vi "NI6071E.ProcCases.vi"(0 "i ref in":refnum<vi>, 1 "selector":string, 2 "data":i8[](array[numeric]), 3 "call cluster":T4={"Object"="", "Selector"="", "CallType"=enum."synchronous", "Async Object"="", "Async Selector"="", "Data Descriptor"="", "Data"=[], "Error #"=0, "Expire"=0}, 5 "error in":errorcluster) -> (14 "i ref out":refnum<vi>, 17 "answer cluster":T4={"Object"="", "Selector"="", "CallType"=enum."synchronous", "Async Object"="", "Async Selector"="", "Data Descriptor"="", "Data"=[], "Error #"=0, "Expire"=0}, 19 "error out":errorcluster)   [LabVIEW 2014, in "NI6071E.lvlib"]
doc: "This method is called by a process from within the default case in the event loop. The methods of a class that are linked to events will be called from THIS method. Add your code here."
uses:
  NI6071E.lvlib
  CSCore/CSSystem/CoreDefs/CoreDefs.call_type.ctl
  CSCore/BaseProcess/BaseProcess.descriptor string definition.ctl
  CSCore/CSSystem/CoreDefs/CoreDefs.rawDataType.ctl
  NI6071EConfig.ctl
  NI6071EStart.ctl
  NI6071ERead.ctl
  CSCore/CSSystem/CoreLib/CoreLib.byte array 2 string.vi
  CSCore/CSSystem/CoreLib/CoreLib.byte array 2 int.vi
  CSCore/CSSystem/CoreLib/CoreLib.string 2 byte array.vi
  CSCore/BaseProcess/BaseProcess.lvlib
  CSCore/CSSystem/CoreLib/CoreLib.lvlib
panel:
  in  "NI6071E Read":T1={"time limit in sec (-1:auto calculate)"=-1.0, "number of scans to read (-1:all)"=-1} {"time limit in sec (-1:auto calculate)" format="%0.2f"}
  in  "NI6071E Start":T2={"scan rate (40000 scans/sec)"=1000.0, "trigger type (analog)"=enum."no trigger", "edge or slope \n(rising)"=enum."rising", "number of buffers to acquire (1)"=1, "analog chan (PFI0) & level (2.00)"={"trigger channel (empty)"="", "level (0.0)"=0.0}, "[additional trig params]"={"hysteresis (0.0)"=-1.0, "coupling (no change:0)"=enum."no change", "delay (0 sec)"=0.0, "skip count (0)"=0, "time limit (0 sec)"=0.0}} {"[additional trig params]"."time limit (0 sec)" format="%0.2f"; "[additional trig params]"."delay (0 sec)" format="%0.2f"; "[additional trig params]"."hysteresis (0.0)" format="%0.2f"; "analog chan (PFI0) & level (2.00)"."level (0.0)" format="%0.2f"; "scan rate (40000 scans/sec)" format="%0.2f"}
  in  "NI6071E Config":T3={"device (1)"=5, "channels (0)"=["0", "1", "2"], "buffer size (1000 scans)"=1000, "[number of buffers] (1)"=1, "measurement mode structure"={"measurement mode"=0, "reserved"=0}, "input limits (no change)"=[], "coupling & input config (no change:0)"=[]} {"measurement mode structure"."measurement mode" items=["no change", "Volts", "Volts RMS", "Ohms", "Diode", "4-wire ohms", "Current", "Current RMS"]; "coupling & input config (no change:0)"."input config (no change:0)" items=["no change", "differential", "ref. single-ended", "non-ref. single-ended", "4-wire"]; "input limits (no change)"."low limit (0.0)" format="%0.2f"; "input limits (no change)"."high limit (0.0)" format="%0.2f"}
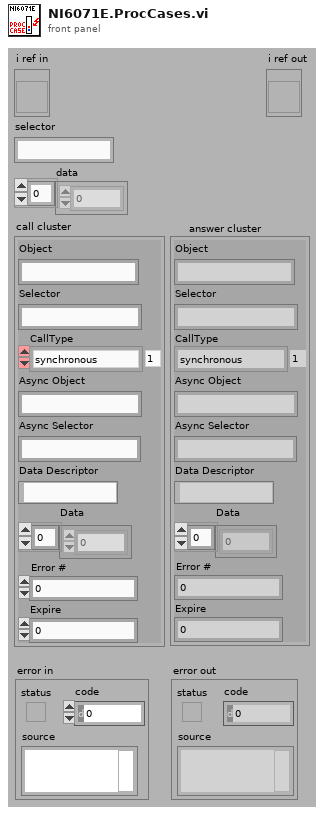
[diagram p1: front panel]
types:
  T1 = typedef "NI6071E.lvlib/NI6071ERead.ctl" = cluster{"time limit in sec (-1:auto calculate)":sgl, "number of scans to read (-1:all)":i32}
  T2 = typedef "NI6071E.lvlib/NI6071EStart.ctl" = cluster{"scan rate (40000 scans/sec)":sgl, "trigger type (analog)":enum16{"no trigger", "analog", "digital A", "digital A & B", "scan clock gate"}, "edge or slope \n(rising)":enum16{"no change", "rising", "falling"}, "number of buffers to acquire (1)":i32, "analog chan (PFI0) & level (2.00)":cluster{"trigger channel (empty)":string, "level (0.0)":sgl}, "[additional trig params]":cluster{"hysteresis (0.0)":sgl, "coupling (no change:0)":enum16{"no change", "DC", "AC"}, "delay (0 sec)":sgl, "skip count (0)":i32, "time limit (0 sec)":sgl}}
  T3 = typedef "NI6071E.lvlib/NI6071EConfig.ctl" = cluster{"device (1)":i16, "channels (0)":tag[], "buffer size (1000 scans)":i32, "[number of buffers] (1)":i32, "measurement mode structure":cluster{"measurement mode":u16, "reserved":u32}, "input limits (no change)":cluster{"high limit (0.0)":sgl, "low limit (0.0)":sgl}[], "coupling & input config (no change:0)":cluster{"coupling (no change:0)":enum16{"no change", "DC", "AC", "GND", "internal ref."}, "input config (no change:0)":u16}[]}
  T4 = typedef "CoreDefs.call_type.ctl" = cluster{"Object":string, "Selector":string, "CallType":enum16{"simple", "synchronous", "asynchronous"}, "Async Object":string, "Async Selector":string, "Data Descriptor":T5, "Data":T6, "Error #":i32, "Expire":u32}
  T5 = typedef "BaseProcess.lvlib/BaseProcess.descriptor string definition.ctl" = string
  T6 = typedef "CoreDefs.rawDataType.ctl" = i8[]
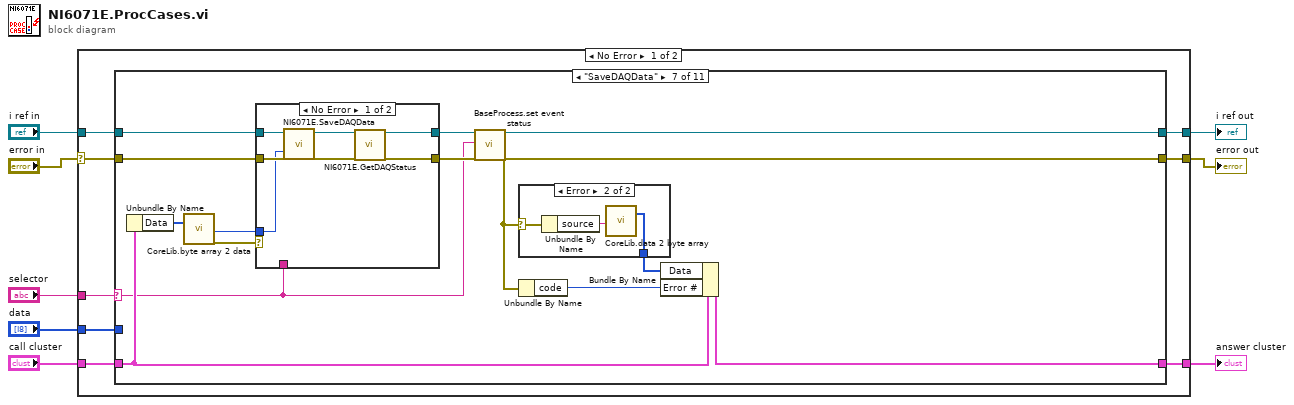
[diagram p0: block diagram]
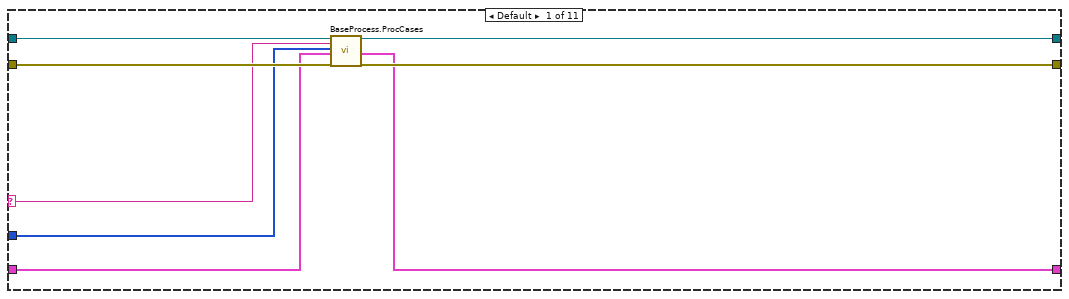
[diagram p2: hidden frame]
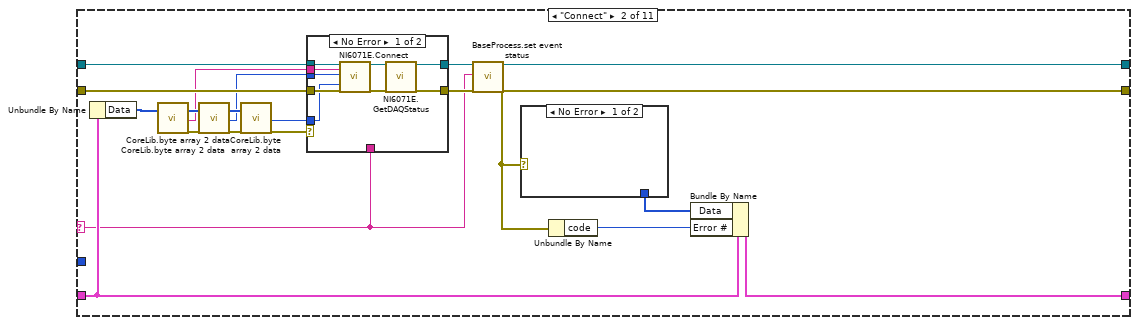
[diagram p3: hidden frame]
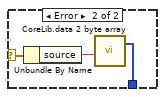
[diagram p4: hidden frame]
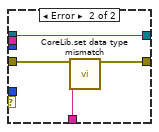
[diagram p5: hidden frame]
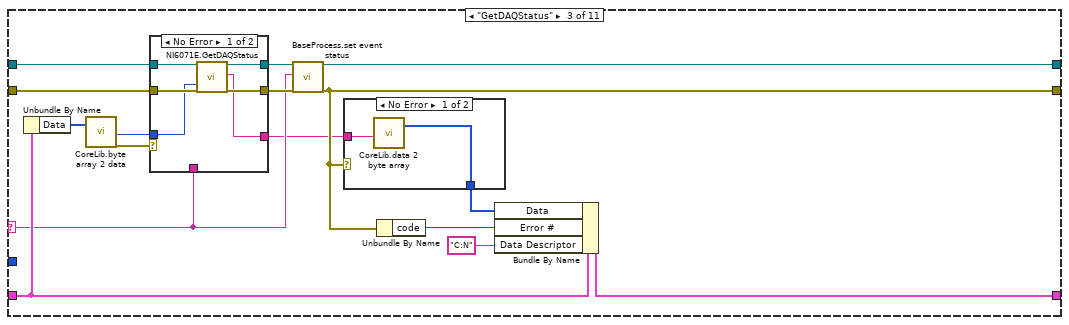
[diagram p6: hidden frame]
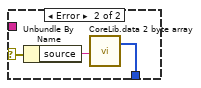
[diagram p7: hidden frame]
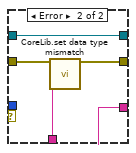
[diagram p8: hidden frame]
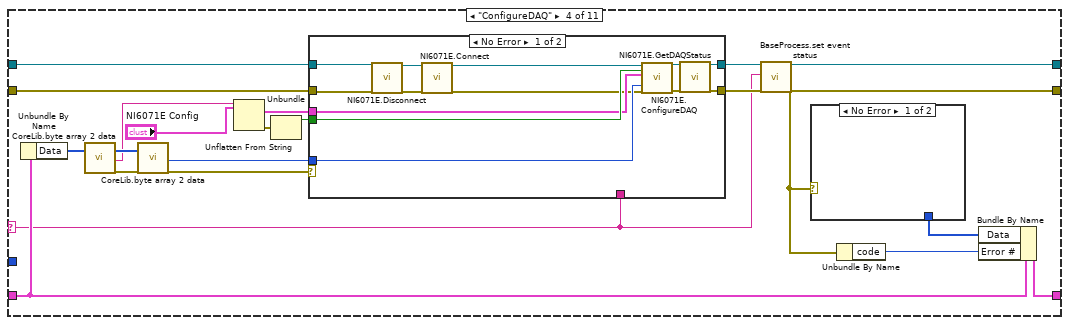
[diagram p9: hidden frame]
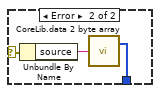
[diagram p10: hidden frame]
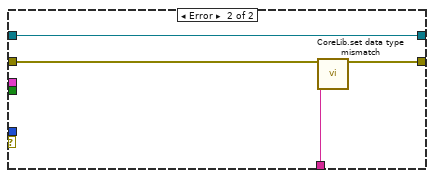
[diagram p11: hidden frame]
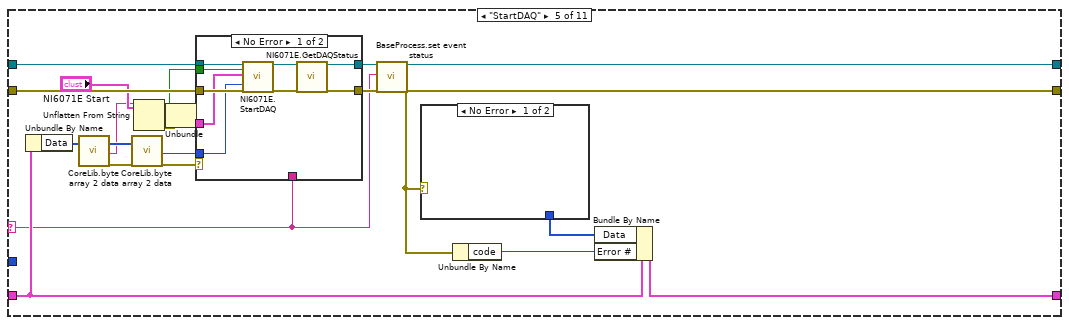
[diagram p12: hidden frame]
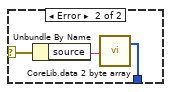
[diagram p13: hidden frame]
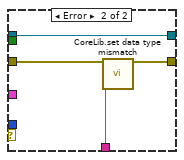
[diagram p14: hidden frame]
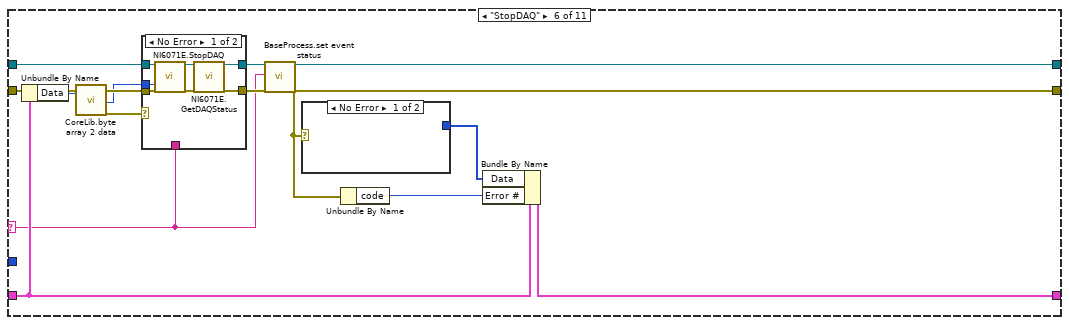
[diagram p15: hidden frame]
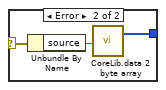
[diagram p16: hidden frame]
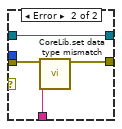
[diagram p17: hidden frame]
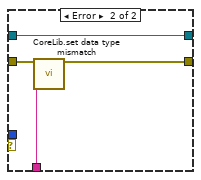
[diagram p19: hidden frame]
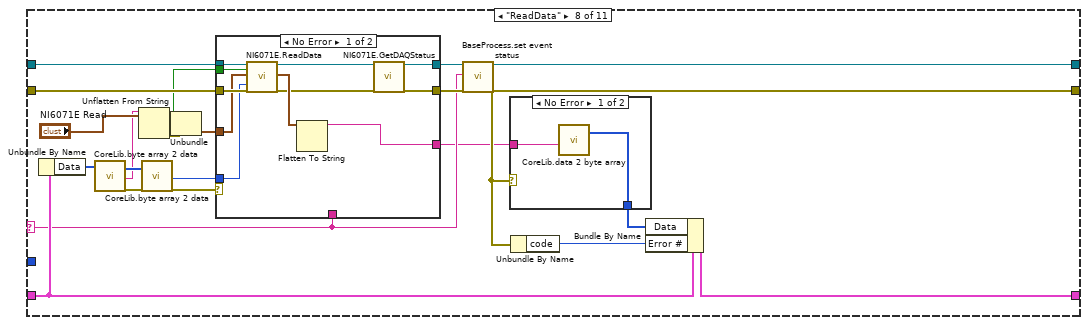
[diagram p20: hidden frame]
diagram:
  n1 = case shown="No Error" "error in" {
    selector: "error in" -> [w9 w352]
    tunnel: "selector" -> [w16 _]
    tunnel: [w15 w353] -> w7
    tunnel: "call cluster" -> [w14 w353]
    tunnel: "i ref in" -> [w13 w354]
    tunnel: [w12 w354] -> w4
    tunnel: [w11 w352] -> w3
    tunnel: "data" -> [w10 _]
    frame No Error {
      n2 = case shown="\"SaveDAQData\"" w16 {
        selector: w16 -> [w19 w36 w68 w105 w146 w176 w204 w240 w276 w310 w339]
        tunnel: w13 -> [w18 w44 w76 w113 w154 w184 w212 w248 w284 w318 w342]
        tunnel: [w24 w35 w67 w104 w145 w175 w203 w239 w275 w309 w344] -> w12
        tunnel: w14 -> [w20 w41 w73 w110 w151 w181 w209 w245 w281 w315 w347]
        tunnel: [w21 w40 w72 w109 w150 w180 w208 w244 w280 w314 w346] -> w15
        tunnel: w9 -> [w23 w43 w75 w112 w153 w183 w211 w247 w283 w317 w341]
        tunnel: [w22 w37 w69 w106 w147 w177 w205 w241 w277 w311 w345] -> w11
        tunnel: w10 -> [w17 _ _ _ _ _ _ _ _ _ _]
        frame Default {
          n3 = call "BaseProcess.ProcCases.vi"("i ref in"=w18, "selector"=w19, "Data"=w17, "call cluster"=w20, "error in (no error)"=w23) -> ("i ref out"=w24:refnum<vi>, "answer cluster"=w21:T4, "error out"=w22:errorcluster)  [unwired: 12 in]
        }
        frame "Connect" {
          n4 = Unbundle By Name(w41) -> ("Data"=w29:T6)
          n5 = call-poly "CoreLib.byte array 2 data.vi"("byteArray"=w29) -> ("byteArray out"=w33:T6, "string"=w28:string, "error out"=w32:errorcluster)  [unwired: 16 in]
          n6 = call-poly "CoreLib.byte array 2 data.vi"("byteArray"=w33, "error in (no error)"=w32) -> ("byteArray out"=w31:T6, "i32"=w27:i32, "error out"=w30:errorcluster)  [unwired: 15 in]
          n7 = call-poly "CoreLib.byte array 2 data.vi"("byteArray"=w31, "error in (no error)"=w30) -> ("i32"=w26:i32, "error out"=w25:errorcluster)  [unwired: 15 in, 1 out]
          n8 = case shown="No Error" w25 {
            tunnel: [w50 w60] -> w39
            tunnel: w44 -> [w55 w60]
            tunnel: w43 -> [w54 w59]
            tunnel: [w48 w58] -> w38
            tunnel: w27 -> [w56 _]
            tunnel: w36 -> [_ w57]
            tunnel: w28 -> [w53 _]
            tunnel: w26 -> [w52 _]
            frame No Error {
              n9 = call "NI6071E.Connect.vi"("i ref in"=w55, "Node name"=w53, "Port"=w56, "timeout ms (60000)"=w52, "error in (no error)"=w54) -> ("i ref out"=w51:refnum<vi>, "error out"=w49:errorcluster)  [unwired: 13 in]
              n10 = call "NI6071E.GetDAQStatus.vi"("i ref in"=w51, "error in (no error)"=w49) -> ("i ref out"=w50:refnum<vi>, "error out"=w48:errorcluster)  [unwired: 15 in, 1 out]
            }
            frame Error {
              n11 = call "CoreLib.set data type mismatch.vi"("error in (no error)"=w59, "error source"=w57) -> ("error out"=w58:errorcluster)  [unwired: 17 in]
            }
          }
          n12 = call "BaseProcess.set event status.vi"("i ref in"=w39, "EventStatus"=w36, "error in (no error)"=w38) -> ("i ref out"=w35:refnum<vi>, "error out"=w37:errorcluster)  [unwired: 14 in, 1 out]
          n13 = case shown="No Error" w37 {
            selector: w37 -> [_ w47]
            tunnel: [_ w45] -> w34
            frame No Error {
            }
            frame Error {
              n14 = Unbundle By Name(w47) -> ("source"=w46:string)
              n15 = call-poly "CoreLib.data 2 byte array.vi"("string"=w46) -> ("byteArray out"=w45:T6)  [unwired: 18 in]
            }
          }
          n16 = Unbundle By Name(w37) -> ("code"=w42:i32)
          n17 = Bundle By Name(cluster=w41, "Data"=w34, "Error #"=w42) -> (w40:T4)
        }
        frame "GetDAQStatus" {
          n18 = Unbundle By Name(w73) -> ("Data"=w63:T6)
          n19 = call-poly "CoreLib.byte array 2 data.vi"("byteArray"=w63) -> ("i32"=w62:i32, "error out"=w61:errorcluster)  [unwired: 16 in, 1 out]
          n20 = case shown="No Error" w61 {
            tunnel: [w86 w92] -> w71
            tunnel: w76 -> [w87 w92]
            tunnel: w75 -> [w85 w91]
            tunnel: [w84 w90] -> w70
            tunnel: w68 -> [_ w89]
            tunnel: w62 -> [w83 _]
            tunnel: [w82 "" ("Status")] -> w65
            frame No Error {
              n21 = call "NI6071E.GetDAQStatus.vi"("i ref in"=w87, "timeout ms (60000)"=w83, "error in (no error)"=w85) -> ("i ref out"=w86:refnum<vi>, "Status"=w82:string, "error out"=w84:errorcluster)  [unwired: 14 in]
            }
            frame Error {
              n22 = call "CoreLib.set data type mismatch.vi"("error in (no error)"=w91, "error source"=w89) -> ("error out"=w90:errorcluster)  [unwired: 17 in]
            }
          }
          n23 = call "BaseProcess.set event status.vi"("i ref in"=w71, "EventStatus"=w68, "error in (no error)"=w70) -> ("i ref out"=w67:refnum<vi>, "error out"=w69:errorcluster)  [unwired: 14 in, 1 out]
          n24 = case shown="No Error" w69 {
            selector: w69 -> [_ w81]
            tunnel: w65 -> [w78 _]
            tunnel: [w77 w79] -> w64
            frame No Error {
              n25 = call-poly "CoreLib.data 2 byte array.vi"("string"=w78) -> ("byteArray out"=w77:T6)  [unwired: 18 in]
            }
            frame Error {
              n26 = Unbundle By Name(w81) -> ("source"=w80:string)
              n27 = call-poly "CoreLib.data 2 byte array.vi"("string"=w80) -> ("byteArray out"=w79:T6)  [unwired: 18 in]
            }
          }
          n28 = Unbundle By Name(w69) -> ("code"=w74:i32)
          n29 = Bundle By Name(cluster=w73, "Data"=w64, "Error #"=w74, "Data Descriptor"="C:N") -> (w72:T4)
        }
        frame "ConfigureDAQ" {
          n30 = Unbundle By Name(w110) -> ("Data"=w96:T6)
          n31 = call-poly "CoreLib.byte array 2 data.vi"("byteArray"=w96) -> ("byteArray out"=w100:T6, "string"=w98:string, "error out"=w99:errorcluster)  [unwired: 16 in]
          n32 = call-poly "CoreLib.byte array 2 data.vi"("byteArray"=w100, "error in (no error)"=w99) -> ("i32"=w97:i32, "error out"=w95:errorcluster)  [unwired: 15 in, 1 out]
          n33 = Unflatten From String(type="NI6071E Config", binary string=w98) -> (value=w102:T3, error out=w93:errorcluster)  [unwired: 3 in, 1 out]
          n34 = Unbundle(w93) -> ("status"=w101:bool)  [unwired: 2 out]
          n35 = case shown="No Error" w95 {
            tunnel: [w125 w133] -> w108
            tunnel: w113 -> [w121 w133]
            tunnel: w112 -> [w122 w132]
            tunnel: [w123 w130] -> w107
            tunnel: w97 -> [w127 _]
            tunnel: w105 -> [_ w131]
            tunnel: w102 -> [w128 _]
            tunnel: w101 -> [w129 _]
            frame No Error {
              n36 = call "NI6071E.Disconnect.vi"("i ref in"=w121, "error in (no error)"=w122) -> ("i ref out"=w120:refnum<vi>, "error out"=w118:errorcluster)  [unwired: 16 in]
              n37 = call "NI6071E.Connect.vi"("i ref in"=w120, "error in (no error)"=w118) -> ("i ref out"=w119:refnum<vi>, "error out"=w117:errorcluster)  [unwired: 16 in]
              n38 = call "NI6071E.ConfigureDAQ.vi"("i ref in"=w119, "Use attribute data (f)"=w129, "NI6071E Config"=w128, "timeout ms (60000)"=w127, "error in (no error)"=w117) -> ("i ref out"=w126:refnum<vi>, "error out"=w124:errorcluster)  [unwired: 13 in]
              n39 = call "NI6071E.GetDAQStatus.vi"("i ref in"=w126, "error in (no error)"=w124) -> ("i ref out"=w125:refnum<vi>, "error out"=w123:errorcluster)  [unwired: 15 in, 1 out]
            }
            frame Error {
              n40 = call "CoreLib.set data type mismatch.vi"("error in (no error)"=w132, "error source"=w131) -> ("error out"=w130:errorcluster)  [unwired: 17 in]
            }
          }
          n41 = call "BaseProcess.set event status.vi"("i ref in"=w108, "EventStatus"=w105, "error in (no error)"=w107) -> ("i ref out"=w104:refnum<vi>, "error out"=w106:errorcluster)  [unwired: 14 in, 1 out]
          n42 = case shown="No Error" w106 {
            selector: w106 -> [_ w116]
            tunnel: [_ w114] -> w94
            frame No Error {
            }
            frame Error {
              n43 = Unbundle By Name(w116) -> ("source"=w115:string)
              n44 = call-poly "CoreLib.data 2 byte array.vi"("string"=w115) -> ("byteArray out"=w114:T6)  [unwired: 18 in]
            }
          }
          n45 = Unbundle By Name(w106) -> ("code"=w111:i32)
          n46 = Bundle By Name(cluster=w110, "Data"=w94, "Error #"=w111) -> (w109:T4)
        }
        frame "StartDAQ" {
          n47 = Unbundle By Name(w151) -> ("Data"=w139:T6)
          n48 = call-poly "CoreLib.byte array 2 data.vi"("byteArray"=w139) -> ("byteArray out"=w140:T6, "string"=w138:string, "error out"=w141:errorcluster)  [unwired: 16 in]
          n49 = call-poly "CoreLib.byte array 2 data.vi"("byteArray"=w140, "error in (no error)"=w141) -> ("i32"=w137:i32, "error out"=w136:errorcluster)  [unwired: 15 in, 1 out]
          n50 = Unflatten From String(type="NI6071E Start", binary string=w138) -> (value=w143:T2, error out=w134:errorcluster)  [unwired: 3 in, 1 out]
          n51 = Unbundle(w134) -> ("status"=w142:bool)  [unwired: 2 out]
          n52 = case shown="No Error" w136 {
            tunnel: [w158 w170] -> w149
            tunnel: w154 -> [w166 w170]
            tunnel: w153 -> [w165 w169]
            tunnel: [w160 w168] -> w148
            tunnel: w137 -> [w162 _]
            tunnel: w146 -> [_ w167]
            tunnel: w143 -> [w163 _]
            tunnel: w142 -> [w164 _]
            frame No Error {
              n53 = call "NI6071E.StartDAQ.vi"("i ref in"=w166, "Use attribute data (f)"=w164, "PPMA DAQ Start"=w163, "timeout ms (60000)"=w162, "error in (no error)"=w165) -> ("i ref out"=w159:refnum<vi>, "error out"=w161:errorcluster)  [unwired: 13 in]
              n54 = call "NI6071E.GetDAQStatus.vi"("i ref in"=w159, "error in (no error)"=w161) -> ("i ref out"=w158:refnum<vi>, "error out"=w160:errorcluster)  [unwired: 15 in, 1 out]
            }
            frame Error {
              n55 = call "CoreLib.set data type mismatch.vi"("error in (no error)"=w169, "error source"=w167) -> ("error out"=w168:errorcluster)  [unwired: 17 in]
            }
          }
          n56 = call "BaseProcess.set event status.vi"("i ref in"=w149, "EventStatus"=w146, "error in (no error)"=w148) -> ("i ref out"=w145:refnum<vi>, "error out"=w147:errorcluster)  [unwired: 14 in, 1 out]
          n57 = case shown="No Error" w147 {
            selector: w147 -> [_ w157]
            tunnel: [_ w156] -> w135
            frame No Error {
            }
            frame Error {
              n58 = Unbundle By Name(w157) -> ("source"=w155:string)
              n59 = call-poly "CoreLib.data 2 byte array.vi"("string"=w155) -> ("byteArray out"=w156:T6)  [unwired: 18 in]
            }
          }
          n60 = Unbundle By Name(w147) -> ("code"=w152:i32)
          n61 = Bundle By Name(cluster=w151, "Data"=w135, "Error #"=w152) -> (w150:T4)
        }
        frame "StopDAQ" {
          n62 = Unbundle By Name(w181) -> ("Data"=w174:T6)
          n63 = call-poly "CoreLib.byte array 2 data.vi"("byteArray"=w174) -> ("i32"=w173:i32, "error out"=w172:errorcluster)  [unwired: 16 in, 1 out]
          n64 = case shown="No Error" w172 {
            tunnel: [w189 w198] -> w179
            tunnel: w184 -> [w194 w198]
            tunnel: w183 -> [w193 w197]
            tunnel: [w190 w196] -> w178
            tunnel: w173 -> [w192 _]
            tunnel: w176 -> [_ w195]
            frame No Error {
              n65 = call "NI6071E.StopDAQ.vi"("i ref in"=w194, "timeout ms (60000)"=w192, "error in (no error)"=w193) -> ("i ref out"=w188:refnum<vi>, "error out"=w191:errorcluster)  [unwired: 15 in]
              n66 = call "NI6071E.GetDAQStatus.vi"("i ref in"=w188, "error in (no error)"=w191) -> ("i ref out"=w189:refnum<vi>, "error out"=w190:errorcluster)  [unwired: 15 in, 1 out]
            }
            frame Error {
              n67 = call "CoreLib.set data type mismatch.vi"("error in (no error)"=w197, "error source"=w195) -> ("error out"=w196:errorcluster)  [unwired: 17 in]
            }
          }
          n68 = call "BaseProcess.set event status.vi"("i ref in"=w179, "EventStatus"=w176, "error in (no error)"=w178) -> ("i ref out"=w175:refnum<vi>, "error out"=w177:errorcluster)  [unwired: 14 in, 1 out]
          n69 = case shown="No Error" w177 {
            selector: w177 -> [_ w187]
            tunnel: [_ w185] -> w171
            frame No Error {
            }
            frame Error {
              n70 = Unbundle By Name(w187) -> ("source"=w186:string)
              n71 = call-poly "CoreLib.data 2 byte array.vi"("string"=w186) -> ("byteArray out"=w185:T6)  [unwired: 18 in]
            }
          }
          n72 = Unbundle By Name(w177) -> ("code"=w182:i32)
          n73 = Bundle By Name(cluster=w181, "Data"=w171, "Error #"=w182) -> (w180:T4)
        }
        frame "SaveDAQData" {
          n74 = Unbundle By Name(w209) -> ("Data"=w202:T6)
          n75 = call-poly "CoreLib.byte array 2 data.vi"("byteArray"=w202) -> ("i32"=w201:i32, "error out"=w200:errorcluster)  [unwired: 16 in, 1 out]
          n76 = case shown="No Error" w200 {
            tunnel: [w218 w226] -> w207
            tunnel: w212 -> [w222 w226]
            tunnel: w211 -> [w221 w225]
            tunnel: [w216 w224] -> w206
            tunnel: w201 -> [w220 _]
            tunnel: w204 -> [_ w223]
            frame No Error {
              n77 = call "NI6071E.SaveDAQData.vi"("i ref in"=w222, "timeout ms (60000)"=w220, "error in (no error)"=w221) -> ("i ref out"=w219:refnum<vi>, "error out"=w217:errorcluster)  [unwired: 15 in]
              n78 = call "NI6071E.GetDAQStatus.vi"("i ref in"=w219, "error in (no error)"=w217) -> ("i ref out"=w218:refnum<vi>, "error out"=w216:errorcluster)  [unwired: 15 in, 1 out]
            }
            frame Error {
              n79 = call "CoreLib.set data type mismatch.vi"("error in (no error)"=w225, "error source"=w223) -> ("error out"=w224:errorcluster)  [unwired: 17 in]
            }
          }
          n80 = call "BaseProcess.set event status.vi"("i ref in"=w207, "EventStatus"=w204, "error in (no error)"=w206) -> ("i ref out"=w203:refnum<vi>, "error out"=w205:errorcluster)  [unwired: 14 in, 1 out]
          n81 = case shown="Error" w205 {
            selector: w205 -> [_ w215]
            tunnel: [_ w214] -> w199
            frame No Error {
            }
            frame Error {
              n82 = Unbundle By Name(w215) -> ("source"=w213:string)
              n83 = call-poly "CoreLib.data 2 byte array.vi"("string"=w213) -> ("byteArray out"=w214:T6)  [unwired: 18 in]
            }
          }
          n84 = Unbundle By Name(w205) -> ("code"=w210:i32)
          n85 = Bundle By Name(cluster=w209, "Data"=w199, "Error #"=w210) -> (w208:T4)
        }
        frame "ReadData" {
          n86 = Unbundle By Name(w245) -> ("Data"=w231:T6)
          n87 = call-poly "CoreLib.byte array 2 data.vi"("byteArray"=w231) -> ("byteArray out"=w233:T6, "string"=w229:string, "error out"=w232:errorcluster)  [unwired: 16 in]
          n88 = Unflatten From String(type="NI6071E Read", binary string=w229) -> (value=w237:T1, error out=w227:errorcluster)  [unwired: 3 in, 1 out]
          n89 = call-poly "CoreLib.byte array 2 data.vi"("byteArray"=w233, "error in (no error)"=w232) -> ("i32"=w230:i32, "error out"=w228:errorcluster)  [unwired: 15 in, 1 out]
          n90 = Unbundle(w227) -> ("status"=w236:bool)  [unwired: 2 out]
          n91 = case shown="No Error" w228 {
            tunnel: [w256 w269] -> w243
            tunnel: w248 -> [w263 w269]
            tunnel: w247 -> [w262 w268]
            tunnel: [w254 w267] -> w242
            tunnel: w230 -> [w261 _]
            tunnel: w240 -> [_ w266]
            tunnel: w237 -> [w260 _]
            tunnel: [w264 "" ("data string")] -> w235
            tunnel: w236 -> [w259 _]
            frame No Error {
              n92 = call "NI6071E.ReadData.vi"("i ref in"=w263, "Use attribute data (f)"=w259, "NI6071E Read"=w260, "timeout ms (60000)"=w261, "error in (no error)"=w262) -> ("i ref out"=w257:refnum<vi>, "Waveforms"=w258:waveform(dbl)[], "error out"=w255:errorcluster)  [unwired: 12 in]
              n93 = Flatten To String(anything=w258) -> (data string=w264:string)  [unwired: 3 in, 2 out]
              n94 = call "NI6071E.GetDAQStatus.vi"("i ref in"=w257, "error in (no error)"=w255) -> ("i ref out"=w256:refnum<vi>, "error out"=w254:errorcluster)  [unwired: 15 in, 1 out]
            }
            frame Error {
              n95 = call "CoreLib.set data type mismatch.vi"("error in (no error)"=w268, "error source"=w266) -> ("error out"=w267:errorcluster)  [unwired: 17 in]
            }
          }
          n96 = call "BaseProcess.set event status.vi"("i ref in"=w243, "EventStatus"=w240, "error in (no error)"=w242) -> ("i ref out"=w239:refnum<vi>, "error out"=w241:errorcluster)  [unwired: 14 in, 1 out]
          n97 = case shown="No Error" w241 {
            selector: w241 -> [_ w253]
            tunnel: w235 -> [w250 _]
            tunnel: [w249 w251] -> w234
            frame No Error {
              n98 = call-poly "CoreLib.data 2 byte array.vi"("string"=w250) -> ("byteArray out"=w249:T6)  [unwired: 18 in]
            }
            frame Error {
              n99 = Unbundle By Name(w253) -> ("source"=w252:string)
              n100 = call-poly "CoreLib.data 2 byte array.vi"("string"=w252) -> ("byteArray out"=w251:T6)  [unwired: 18 in]
            }
          }
          n101 = Unbundle By Name(w241) -> ("code"=w246:i32)
          n102 = Bundle By Name(cluster=w245, "Data"=w234, "Error #"=w246) -> (w244:T4)
        }
        frame "GetWaveform" {
          n103 = Unbundle By Name(w281) -> ("Data"=w270:T6)
          n104 = call-poly "CoreLib.byte array 2 data.vi"("byteArray"=w270) -> ("i32"=w272:i32, "error out"=w271:errorcluster)  [unwired: 16 in, 1 out]
          n105 = case shown="No Error" w271 {
            tunnel: [w291 w303] -> w279
            tunnel: w284 -> [w295 w303]
            tunnel: w283 -> [w297 w302]
            tunnel: [w292 w301] -> w278
            tunnel: w272 -> [w296 _]
            tunnel: w276 -> [_ w300]
            tunnel: [w298 "" ("data string")] -> w274
            frame No Error {
              n106 = call "NI6071E.GetWaveform.vi"("i ref in"=w295, "index"=w296, "error in (no error)"=w297) -> ("i ref out"=w290:refnum<vi>, "Waveform"=w294:waveform(dbl), "error out"=w293:errorcluster)  [unwired: 14 in]
              n107 = Flatten To String(anything=w294) -> (data string=w298:string)  [unwired: 3 in, 2 out]
              n108 = call "NI6071E.GetDAQStatus.vi"("i ref in"=w290, "error in (no error)"=w293) -> ("i ref out"=w291:refnum<vi>, "error out"=w292:errorcluster)  [unwired: 15 in, 1 out]
            }
            frame Error {
              n109 = call "CoreLib.set data type mismatch.vi"("error in (no error)"=w302, "error source"=w300) -> ("error out"=w301:errorcluster)  [unwired: 17 in]
            }
          }
          n110 = call "BaseProcess.set event status.vi"("i ref in"=w279, "EventStatus"=w276, "error in (no error)"=w278) -> ("i ref out"=w275:refnum<vi>, "error out"=w277:errorcluster)  [unwired: 14 in, 1 out]
          n111 = case shown="Error" w277 {
            selector: w277 -> [_ w289]
            tunnel: w274 -> [w286 _]
            tunnel: [w285 w287] -> w273
            frame No Error {
              n112 = call-poly "CoreLib.data 2 byte array.vi"("string"=w286) -> ("byteArray out"=w285:T6)  [unwired: 18 in]
            }
            frame Error {
              n113 = Unbundle By Name(w289) -> ("source"=w288:string)
              n114 = call-poly "CoreLib.data 2 byte array.vi"("string"=w288) -> ("byteArray out"=w287:T6)  [unwired: 18 in]
            }
          }
          n115 = Unbundle By Name(w277) -> ("code"=w282:i32)
          n116 = Bundle By Name(cluster=w281, "Data"=w273, "Error #"=w282) -> (w280:T4)
        }
        frame "GetWaveforms" {
          n117 = Unbundle By Name(w315) -> ("Data"=w307:T6)
          n118 = call-poly "CoreLib.byte array 2 data.vi"("byteArray"=w307) -> ("i32"=w305:i32, "error out"=w306:errorcluster)  [unwired: 16 in, 1 out]
          n119 = case shown="No Error" w306 {
            tunnel: [w324 w337] -> w313
            tunnel: w318 -> [w331 w337]
            tunnel: w317 -> [w330 w336]
            tunnel: [w326 w335] -> w312
            tunnel: w305 -> [w328 _]
            tunnel: w310 -> [_ w334]
            tunnel: [w332 "" ("data string")] -> w304
            frame No Error {
              n120 = call "NI6071E.GetWaveforms.vi"("i ref in"=w331, "ms timeout (-1)"=w328, "error in (no error)"=w330) -> ("i ref out"=w325:refnum<vi>, "Waveforms"=w329:waveform(dbl)[], "error out"=w327:errorcluster)  [unwired: 14 in]
              n121 = call "NI6071E.GetDAQStatus.vi"("i ref in"=w325, "error in (no error)"=w327) -> ("i ref out"=w324:refnum<vi>, "error out"=w326:errorcluster)  [unwired: 15 in, 1 out]
              n122 = Flatten To String(anything=w329) -> (data string=w332:string)  [unwired: 3 in, 2 out]
            }
            frame Error {
              n123 = call "CoreLib.set data type mismatch.vi"("error in (no error)"=w336, "error source"=w334) -> ("error out"=w335:errorcluster)  [unwired: 17 in]
            }
          }
          n124 = call "BaseProcess.set event status.vi"("i ref in"=w313, "EventStatus"=w310, "error in (no error)"=w312) -> ("i ref out"=w309:refnum<vi>, "error out"=w311:errorcluster)  [unwired: 14 in, 1 out]
          n125 = case shown="Error" w311 {
            selector: w311 -> [_ w323]
            tunnel: [w320 w322] -> w308
            tunnel: w304 -> [w319 _]
            frame No Error {
              n126 = call-poly "CoreLib.data 2 byte array.vi"("string"=w319) -> ("byteArray out"=w320:T6)  [unwired: 18 in]
            }
            frame Error {
              n127 = Unbundle By Name(w323) -> ("source"=w321:string)
              n128 = call-poly "CoreLib.data 2 byte array.vi"("string"=w321) -> ("byteArray out"=w322:T6)  [unwired: 18 in]
            }
          }
          n129 = Unbundle By Name(w311) -> ("code"=w316:i32)
          n130 = Bundle By Name(cluster=w315, "Data"=w308, "Error #"=w316) -> (w314:T4)
        }
        frame "Disconnect" {
          n131 = call "NI6071E.Disconnect.vi"("i ref in"=w342, "error in (no error)"=w341) -> ("i ref out"=w343:refnum<vi>, "error out"=w340:errorcluster)  [unwired: 16 in]
          n132 = call "BaseProcess.set event status.vi"("i ref in"=w343, "EventStatus"=w339, "error in (no error)"=w340) -> ("i ref out"=w344:refnum<vi>, "error out"=w345:errorcluster)  [unwired: 14 in, 1 out]
          n133 = case shown="No Error" w345 {
            selector: w345 -> [_ w351]
            tunnel: [_ w349] -> w338
            frame No Error {
            }
            frame Error {
              n134 = Unbundle By Name(w351) -> ("source"=w350:string)
              n135 = call-poly "CoreLib.data 2 byte array.vi"("string"=w350) -> ("byteArray out"=w349:T6)  [unwired: 18 in]
            }
          }
          n136 = Unbundle By Name(w345) -> ("code"=w348:i32)
          n137 = Bundle By Name(cluster=w347, "Data"=w338, "Error #"=w348) -> (w346:T4)
        }
      }
    }
    frame Error {
    }
  }
  "answer cluster" <- w7
  "i ref out" <- w4
  "error out" <- w3
